vi "Untitled 2.vi"() -> ()   [LabVIEW 2024]
panel:
  out "Numeric":i32
  out "Numeric 3":i32
  out "Numeric 2":i32
  # "Fundamentals :"
  # "18~>After running this VI,what is the value displayed in the o/p & iteration count?"
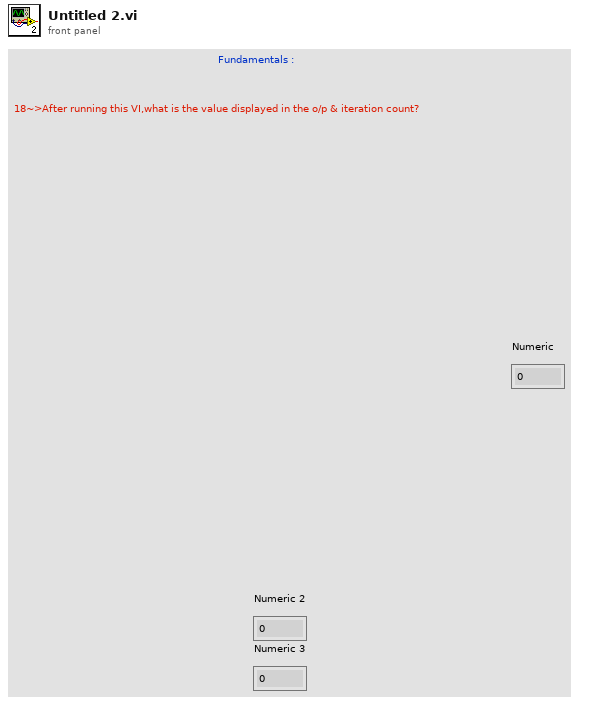
[diagram p1: front panel]
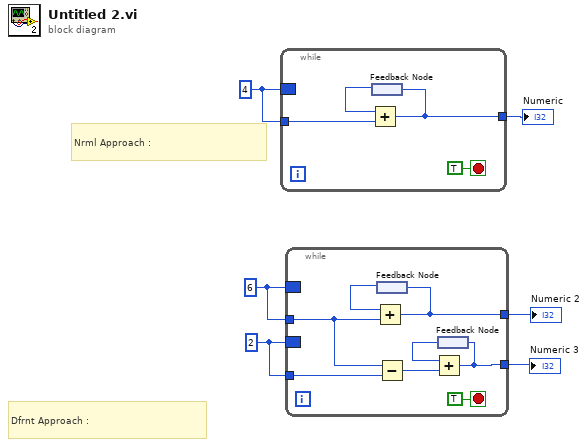
[diagram p0: block diagram]
diagram:
  w2 = 4
  w4 = 2
  w5 = 6
  # "Dfrnt Approach :"
  # "Nrml Approach :"
  n1 = while {
    border: w2 -> [_]
    tunnel: w2 -> [w10]
    tunnel: [w8] -> w1
    stop <- TRUE stop-if-true
    n2 = feedback #1() -> (w9:i32)
    n3 = Add(x=w9, y=w10) -> (x+y=w8:i32)
    n4 = feedback-in #1(w8) -> ()
  }
  "Numeric" <- w1
  n5 = while {
    border: w5 -> [_]
    tunnel: w5 -> [w15]
    tunnel: [w17] -> w6
    border: w4 -> [_]
    tunnel: w4 -> [w14]
    tunnel: [w11] -> w3
    stop <- TRUE stop-if-true
    n6 = feedback #2() -> (w18:i32)
    n7 = Add(x=w18, y=w15) -> (x+y=w17:i32)
    n8 = feedback-in #2(w17) -> ()
    n9 = Subtract(x=w15, y=w14) -> (x-y=w13:i32)
    n10 = feedback #3() -> (w12:i32)
    n11 = Add(x=w12, y=w13) -> (x+y=w11:i32)
    n12 = feedback-in #3(w11) -> ()
  }
  "Numeric 2" <- w6
  "Numeric 3" <- w3
